vi "Action Update Set Point-test-Caraya.vi"(8 "error in (no error)":errorcluster) -> (0 "error out":errorcluster)   [LabVIEW 2018]
uses:
  <vilib>/addons/_JKI Toolkits/Caraya/classes/Assert/Assert True.vi
  <vilib>/addons/_JKI Toolkits/Caraya/classes/Test/Test.lvclass
  Libraries/Thermal Chamber Controller_DQMH/Thermal Chamber Controller_DQMH.lvlib
  <vilib>/addons/_JKI Toolkits/Caraya/classes/Assert/Assert.lvclass
  Libraries/Thermal Chamber Response Simulator/Thermal Chamber Response Simulator.lvlib
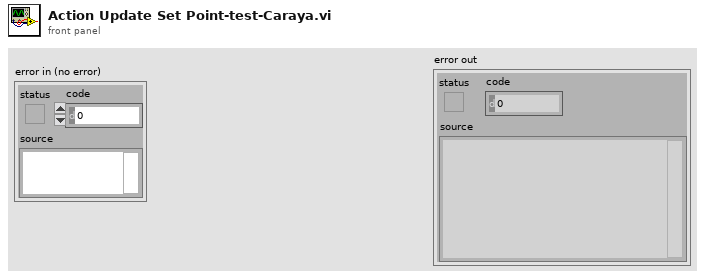
[diagram p1: front panel]
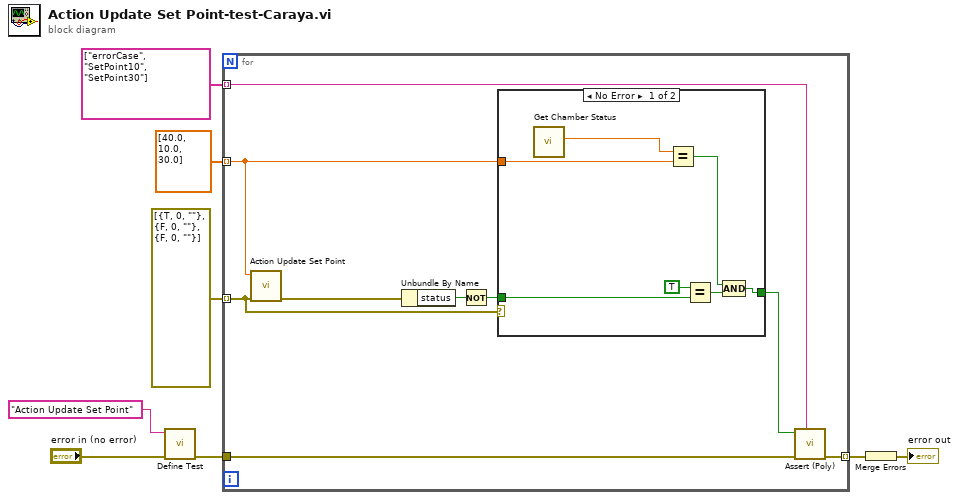
[diagram p0: block diagram]
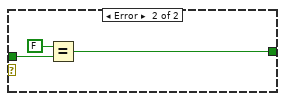
[diagram p2: hidden frame]
diagram:
  n1 = call <vilib>:"Define Test.vi"("error in (no error)"="error in (no error)", "Label (VI Title)"="Action Update Set Point") -> ("error out"=w5:errorcluster)  [unwired: 9 in]
  n2 = for {
    tunnel: string[] ["errorCase", "SetPoint10", "SetPoint30"] -> [w15] mode=indexing
    tunnel: [w17] -> w6 mode=indexing
    tunnel: w5 -> [w16]
    tunnel: dbl[] [40.0, 10.0, 30.0] -> [w9] mode=indexing
    tunnel: errorcluster[] [{"status"=TRUE, "code"=0, "source"=""}, {"status"=FALSE, "code"=0, "source"=""}, {"status"=FALSE, "code"=0, "source"=""}] -> [w10] mode=indexing
    n3 = call "Action Update Set Point.vi"("error in (no error)"=w10, "Temperature Set Point"=w9) -> ("error out"=w13:errorcluster)  [unwired: 9 in]
    n4 = Unbundle By Name(w13) -> ("status"=w14:bool)
    n5 = Not(x=w14) -> (.not. x?=w12:bool)
    n6 = case shown="No Error" w10 {
      tunnel: w12 -> [w19 w26]
      tunnel: [w18 w25] -> w11
      tunnel: w9 -> [w21 _]
      frame No Error {
        n7 = call "Get Chamber Status.vi"() -> ("Temperature Set Point (deg C)"=w20:dbl)  [unwired: 6 in, 5 out]
        n8 = Equal?(x=w20, y=w21) -> (x = y?=w23:bool)
        n9 = Equal?(x=TRUE, y=w19) -> (x = y?=w22:bool)
        n10 = Compound Arithmetic op=AND(w23, w22) -> (w18:bool)
      }
      frame Error {
        n11 = Equal?(x=FALSE, y=w26) -> (x = y?=w25:bool)
      }
    }
    n12 = call-poly <vilib>:"Assert (Poly).vi"("Label"=w15, "error in (no error)"=w16, "True?"=w11) -> ("error out"=w17:errorcluster)  [unwired: 8 in]
  }
  n13 = Merge Errors(w6) -> (→"error out":errorcluster)
